vi "IntParams.vi"(6 "sample interval (s/Pt)":dbl format="%.2f", 7 "prf":dbl=1000.0 format="%.2f", 8 "Length of Subset":i32, 9 "Index of subset":i32, 10 "Data":dbl[](array[numeric]) format="%.2f", 11 "Sens":dbl format="%.2f") -> (3 "Intensity Variables":T1 {"Pulse Int \nIntegral (PII J/cm^2)" format="%.4e"; "Pulse Av Intensity\n (Ipa W/cm^2)" format="%.2f"; "Temporal Av Intensity \n(Ita mW/cm^2)" format="%.2f"; "pulse dur (Pd s)" format="%.2e"})   [LabVIEW 2022 SP3]
uses:
  <vilib>/Analysis/8numeric.llb/1D Numeric Integration.vi
  <vilib>/Analysis/NI_AALPro.lvlib
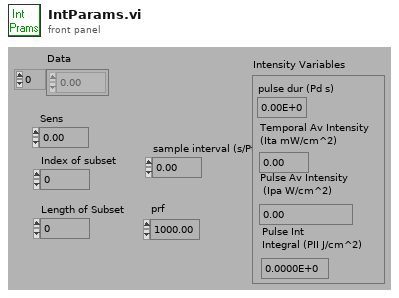
[diagram p1: front panel]
types:
  T1 = cluster{"pulse dur (Pd s)":dbl, "Temporal Av Intensity \n(Ita mW/cm^2)":dbl, "Pulse Av Intensity\n (Ipa W/cm^2)":dbl, "Pulse Int \nIntegral (PII J/cm^2)":dbl}
  T2 = enum32{"Trapezoidal Rule", "Simpson's Rule", "Simpson's 3/8 Rule", "Bode Rule"}
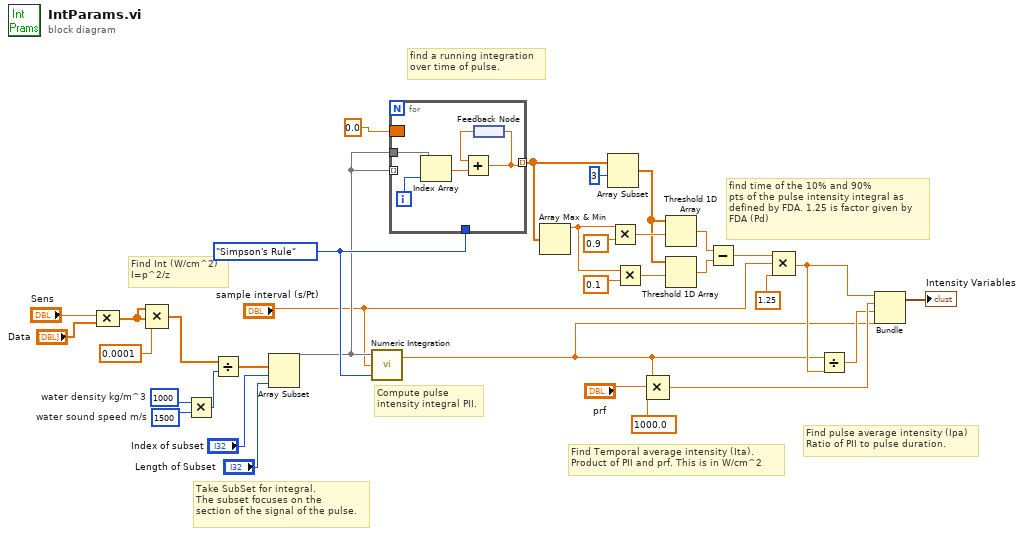
[diagram p0: block diagram]
diagram:
  w20 = 1500  # water sound speed m/s
  w22 = 1000  # water density kg/m^3
  w33 = T2."Simpson's Rule" ("integration method")
  # "Find Temporal average intensity (Ita).\nProduct of PII and prf. This is in W/cm^2"
  # "Find pulse average intensity (Ipa)\nRatio of PII to pulse duration."
  # "Compute pulse\nintensity integral PII."
  # "Find Int (W/cm^2)\nI=p^2/z"
  # "find a running integration\nover time of pulse."
  # "find time of the 10% and 90%\npts of the pulse intensity integral as\ndefined by FDA. 1.25 is factor given by\nFDA (Pd)"
  # "Take SubSet for integral.\nThe subset focuses on the\nsection of the signal of the pulse."
  n1 = Compound Arithmetic op=MULTIPLY("Sens", "Data") -> (w7:dbl[])
  n2 = Compound Arithmetic op=MULTIPLY(w7, w7, 0.0001 ("x")) -> (w9:dbl[])
  n3 = Multiply(x=w22, y=w20) -> (x*y=w21:i32)
  n4 = Divide(x=w9, y=w21) -> (x/y=w19:dbl[])
  n5 = Array Subset(array=w19, index="Index of subset", length="Length of Subset") -> (w4:dbl[])
  n6 = call-poly <vilib>:"Numeric Integration.vi"("integration method"=w33, "dt"="sample interval (s/Pt)", "Input Array"=w4) -> ("result"=w13:dbl)  [unwired: 1 out]
  n7 = for {
    tunnel: w4 -> [w39]
    tunnel: w4 -> [_] mode=indexing
    tunnel: w33 -> [_]
    tunnel: [w35] -> w3 mode=indexing
    border: sgl 0.0 -> [_]
    i -> [w38]
    n8 = Index Array(array=w39, index=w38) -> (element=w36:dbl)
    n9 = feedback #1() -> (w37:dbl)
    n10 = Add(x=w37, y=w36) -> (x+y=w35:dbl)
    n11 = feedback-in #1(w35) -> ()
  }
  n12 = Array Max & Min(array=w3) -> (max value=w2:dbl)  [unwired: 3 out]
  n13 = Array Subset(array=w3, index=3 ("Array Index")) -> (w5:dbl[])  [unwired: 1 in]
  n14 = Multiply(x=w2, y=0.9) -> (x*y=w30:dbl)
  n15 = Multiply(x=w2, y=0.1) -> (x*y=w29:dbl)
  n16 = Compound Arithmetic op=MULTIPLY(w13, "prf", 1000.0 ("x")) -> (w15:dbl)
  n17 = Threshold 1D Array(2:w30, 3:w5) -> (0:w28:dbl)  [unwired: 1 out]
  n18 = Threshold 1D Array(2:w29, 3:w5) -> (0:w27:dbl)  [unwired: 1 out]
  n19 = Subtract(x=w28, y=w27) -> (x-y=w23:dbl)
  n20 = Compound Arithmetic op=MULTIPLY(w23, "sample interval (s/Pt)", 1.25) -> (w16:dbl)
  n21 = Divide(x=w13, y=w16) -> (x/y=w14:dbl)
  n22 = Bundle(w16, w15, w14, "result"=w13) -> (→"Intensity Variables":cluster{dbl, dbl, dbl, "result":dbl})  [unwired: 1 out]
